vi "Get Named Range of Sheet (VAR).vi"(8 "error in":errorcluster, 9 "Sheet Name":string, 10 "Named Range Identifier":string, 11 "SpreadsheetDocument":refnum<k24>) -> (0 "error out":errorcluster, 2 "Cells":variant[][](array[variant]), 3 "SpreadsheetDocument out":refnum<k24>)   [LabVIEW 2021, in "Open Xml.lvlib"]
uses:
  Open Xml.lvlib
  D:/git/Open-Xml-LabVIEW/DocumentFormat.OpenXml.dll
  DocumentFormat.OpenXml.dll
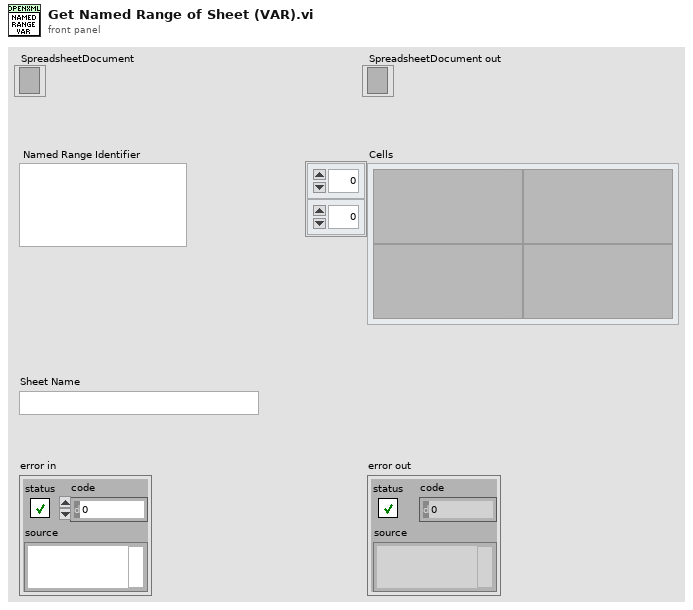
[diagram p1: front panel]
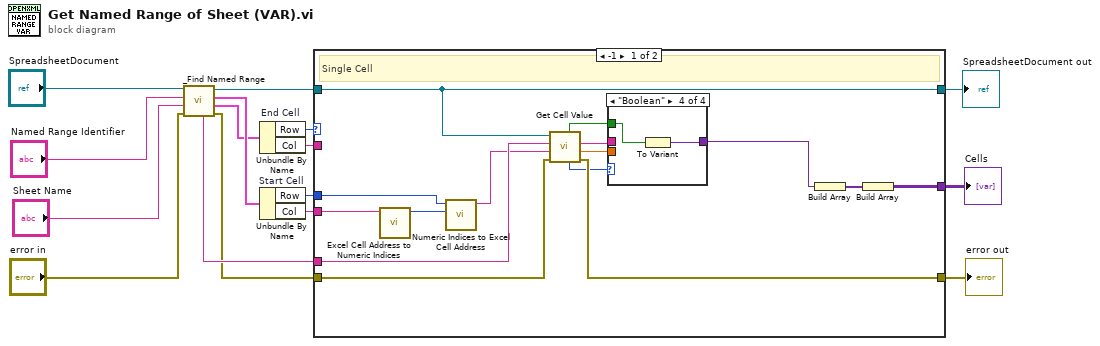
[diagram p0: block diagram]
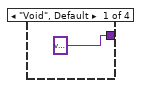
[diagram p2: hidden frame]
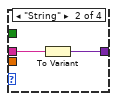
[diagram p3: hidden frame]
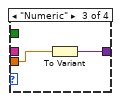
[diagram p4: hidden frame]
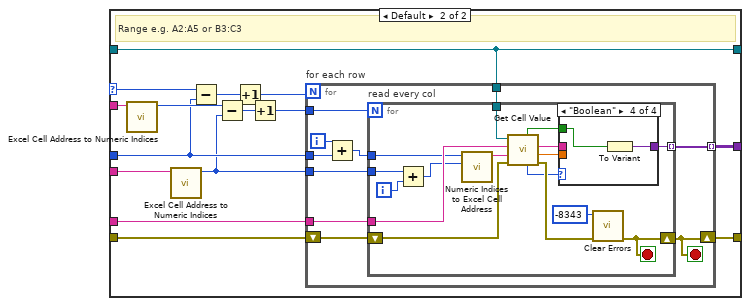
[diagram p5: hidden frame]
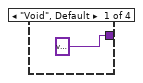
[diagram p6: hidden frame]
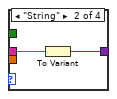
[diagram p7: hidden frame]
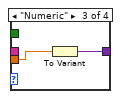
[diagram p8: hidden frame]
diagram:
  n1 = call "_Find Named Range.vi"("error in"="error in", "Sheet Name"="Sheet Name", "Range Identifier"="Named Range Identifier", "SpreadsheetDocument"="SpreadsheetDocument") -> ("error out"=w6:errorcluster, "End Cell"=w14:cluster{"Col":string, "Row":i32}, "Start Cell"=w15:cluster{"Col":string, "Row":i32}, "SpreadsheetDocument"=w3:refnum<k24>, "Sheet Name"=w8:string)  [unwired: 3 in]
  n2 = Unbundle By Name "End Cell"(w14) -> ("Row"=w10:i32, "Col"=w12:string)
  n3 = Unbundle By Name "Start Cell"(w15) -> ("Row"=w9:i32, "Col"=w13:string)
  n4 = case shown="-1" w10 {
    selector: w10 -> [_ w48]
    tunnel: w13 -> [w30 w53]
    tunnel: w12 -> [_ w52]
    tunnel: w9 -> [w22 w45]
    tunnel: w8 -> [w31 w43]
    tunnel: [w24 w42] -> w7
    tunnel: w6 -> [w27 w41]
    tunnel: [w26 w40] -> w5
    tunnel: w3 -> [w23 w39]
    tunnel: [w23 w39] -> w2
    frame -1 {
      # "Single Cell"
      n5 = call "Excel Cell Address to Numeric Indices.vi"("Cell Name"=w30) -> ("Column Number"=w29:i32)  [unwired: 9 in, 1 out]
      n6 = call "Numeric Indices to Excel Cell Address.vi"("Column"=w29, "Row"=w22) -> ("Cell Address"=w28:string)  [unwired: 9 in]
      n7 = call "Get Cell Value.vi"("error in"=w27, "Cell Address"=w28, "Sheet Name"=w31, "SpreadsheetDocument"=w23) -> ("error out"=w26:errorcluster, "Value Numeric"=w18:dbl, "Value String"=w21:string, "Type"=w20:enum16{"Void", "String", "Numeric", "Boolean"}, "Value Boolean"=w17:bool)  [unwired: 2 in, 1 out]
      n8 = case shown="\"Boolean\"" w20 {
        tunnel: w21 -> [_ w34 _ _]
        tunnel: [variant ("Variant") w33 w36 w37] -> w19
        tunnel: w18 -> [_ _ w35 _]
        tunnel: w17 -> [_ _ _ w38]
        frame "Void", Default {
        }
        frame "String" {
          n9 = To Variant(anything=w34) -> (Variant=w33:variant)
        }
        frame "Numeric" {
          n10 = To Variant(anything=w35) -> (Variant=w36:variant)
        }
        frame "Boolean" {
          n11 = To Variant(anything=w38) -> (Variant=w37:variant)
        }
      }
      n12 = Build Array(w19) -> (w25:variant[])
      n13 = Build Array(w25) -> (w24:variant[][])
    }
    frame Default {
      # "Range e.g. A2:A5 or B3:C3"
      n14 = call "Excel Cell Address to Numeric Indices.vi"("Cell Name"=w52) -> ("Column Number"=w51:i32)  [unwired: 9 in, 1 out]
      n15 = call "Excel Cell Address to Numeric Indices.vi"("Cell Name"=w53) -> ("Column Number"=w44:i32)  [unwired: 9 in, 1 out]
      n16 = Subtract(x=w48, y=w45) -> (x-y=w47:i32)
      n17 = Subtract(x=w51, y=w44) -> (x-y=w49:i32)
      n18 = Increment(x=w47) -> (x+1=w46:i32)
      n19 = Increment(x=w49) -> (x+1=w50:i32)
      n20 = for "for each row" {
        N: w46 -> [_]
        tunnel: w50 -> [w63]
        tunnel: w45 -> [w60]
        tunnel: w44 -> [w62]
        tunnel: w43 -> [w61]
        tunnel: [w59] -> w42 mode=indexing
        shift-right: [w55] -> w40
        shift-left: w41 -> [w56]
        tunnel: w39 -> [w54]
        i -> [w57]
        stop <- w55 stop-if-true
        n21 = Add(x=w57, y=w60) -> (x+y=w58:i32)
        n22 = for "read every col" {
          N: w63 -> [_]
          tunnel: w62 -> [w77]
          tunnel: w61 -> [w79]
          tunnel: w58 -> [w76]
          tunnel: [w65] -> w59 mode=indexing
          shift-right: [w71] -> w55
          shift-left: w56 -> [w73]
          tunnel: w54 -> [w69]
          i -> [w74]
          stop <- w71 stop-if-true
          n23 = Add(x=w77, y=w74) -> (x+y=w75:i32)
          n24 = call "Numeric Indices to Excel Cell Address.vi"("Column"=w75, "Row"=w76) -> ("Cell Address"=w78:string)  [unwired: 9 in]
          n25 = call "Get Cell Value.vi"("error in"=w73, "Cell Address"=w78, "Sheet Name"=w79, "SpreadsheetDocument"=w69) -> ("error out"=w72:errorcluster, "Value Numeric"=w67:dbl, "Value String"=w66:string, "Type"=w68:enum16{"Void", "String", "Numeric", "Boolean"}, "Value Boolean"=w64:bool)  [unwired: 2 in, 1 out]
          n26 = case shown="\"Boolean\"" w68 {
            tunnel: w67 -> [_ _ w84 _]
            tunnel: w66 -> [_ w82 _ _]
            tunnel: [variant ("Variant") w81 w83 w86] -> w65
            tunnel: w64 -> [_ _ _ w85]
            frame "Void", Default {
            }
            frame "String" {
              n27 = To Variant(anything=w82) -> (Variant=w81:variant)
            }
            frame "Numeric" {
              n28 = To Variant(anything=w84) -> (Variant=w83:variant)
            }
            frame "Boolean" {
              n29 = To Variant(anything=w85) -> (Variant=w86:variant)
            }
          }
          n30 = call <vilib>:"Clear Errors.vi"("error in (no error)"=w72, "specific error code to clear (0: all)"=-8343) -> ("error out"=w71:errorcluster)  [unwired: 4 in, 1 out]
        }
      }
    }
  }
  "error out" <- w5
  "Cells" <- w7
  "SpreadsheetDocument out" <- w2
